vi "Duplicate String.vi"(10 "Array of Strings":string[](array[string]), 11 "String":string) -> (2 "Exists?":bool, 3 "Updated String":string)   [LabVIEW 2011]
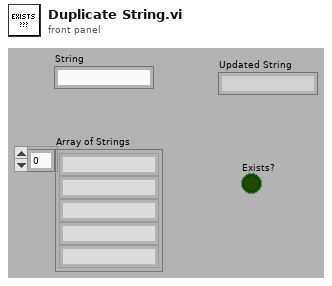
[diagram p1: front panel]
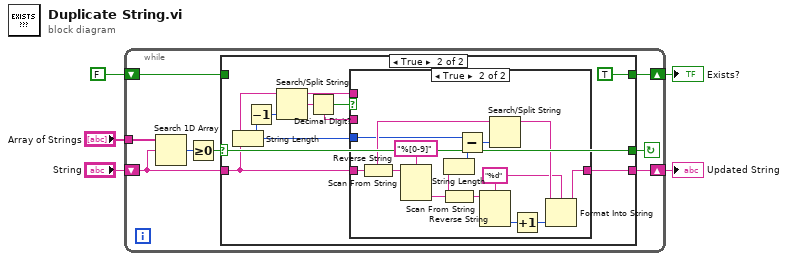
[diagram p0: block diagram]
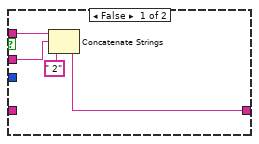
[diagram p3: hidden frame]
diagram:
  n1 = while {
    tunnel: "Array of Strings" -> [w13]
    shift-right: [w10] -> w5
    shift-left: "String" -> [w8]
    shift-right: [w6] -> w2
    shift-left: FALSE -> [w7]
    stop <- w9 continue-if-true
    n2 = Search 1D Array(1D array=w13, element=w8) -> (index of element=w12:i32)  [unwired: 1 out]
    n3 = Greater Or Equal To 0?(x=w12) -> (x >= 0?=w11:bool)
    n4 = case shown="True" w11 {
      selector: w11 -> [w15 w24]
      tunnel: [w15 w24] -> w9
      tunnel: w8 -> [w16 w18]
      tunnel: [w16 w25] -> w10
      tunnel: w7 -> [w14 _]
      tunnel: [w14 TRUE] -> w6
      frame False {
      }
      frame True {
        n5 = String Length(string=w18) -> (length=w17:i32)
        n6 = Decrement(x=w17) -> (x-1=w22:i32)
        n7 = Search/Split String(string=w18, offset (0)=w22) -> (substring before match=w20:string, match + rest of string=w19:string)  [unwired: 2 out]
        n8 = Decimal Digit?(1:w19) -> (0:w21:bool)
        n9 = case shown="True" w21 {
          tunnel: [w27 w42] -> w25
          tunnel: w20 -> [w29 _]
          tunnel: w19 -> [w28 _]
          tunnel: w18 -> [_ w37]
          tunnel: w17 -> [_ w36]
          frame False {
            n10 = Concatenate Strings(w29, w28, " 2") -> (w27:string)
          }
          frame True {
            w32 = "%d"
            n11 = Reverse String(1:w37) -> (0:w40:string)
            n12 = Scan From String(format string="%[0-9]", input string=w40) -> (output 1=w30:string)  [unwired: 2 in, 4 out]
            n13 = String Length(string=w30) -> (length=w35:i32)
            n14 = Reverse String(1:w30) -> (0:w39:string)
            n15 = Subtract(x=w36, y=w35) -> (x-y=w34:i32)
            n16 = Scan From String(format string=w32, input string=w39) -> (output 1=w38:i32)  [unwired: 2 in, 4 out]
            n17 = Search/Split String(string=w37, offset (0)=w34) -> (substring before match=w33:string)  [unwired: 3 out]
            n18 = Increment(x=w38) -> (x+1=w41:i32)
            n19 = Format Into String(format string=w32, initial string=w33, w41) -> (resulting string=w42:string)  [unwired: 1 in, 1 out]
          }
        }
      }
    }
  }
  "Exists?" <- w2
  "Updated String" <- w5
